vi "Process Standard Output.vi"(8 "error in (no error)":errorcluster, 11 "7-zip Wrapper in":refnum<class "7-zip Wrapper.lvclass">) -> (0 "error out":errorcluster, 2 "Command output":string, 3 "7-zip Wrapper out":refnum<class "7-zip Wrapper.lvclass">)   [LabVIEW 2020, in "7-zip Wrapper.lvclass"]
doc: "Process the response for a specific command. Child classes may override this method to process what is returned. The default behavior is to display the whole command response in a dialog box."
uses:
  7-zip Wrapper.lvclass
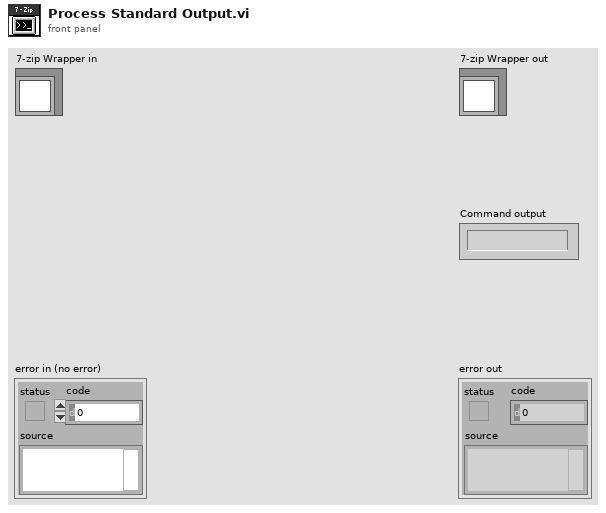
[diagram p1: front panel]
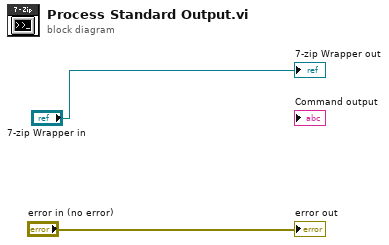
[diagram p0: block diagram]
diagram:
  "error out" <- "error in (no error)"
  "7-zip Wrapper out" <- "7-zip Wrapper in"
